vi "saveDataNodeBegin.vi"(8 "error in (no error)":errorcluster, 9 "indent":i32, 10 "XML Refnum in":refnum<file>, 11 "Category in":refnum<class "Category.lvclass">) -> (0 "error out":errorcluster, 2 "XML Refnum out":refnum<file>, 3 "Category out":refnum<class "Category.lvclass">)   [LabVIEW 2013, in "Category.lvclass"]
doc: "Begins the process of saving a xceData Node to an XML formatted file."
uses:
  Category.lvclass
  xCE/xceDataNode/xceDataNode.lvclass
  Category.lvclass/Category.ctl
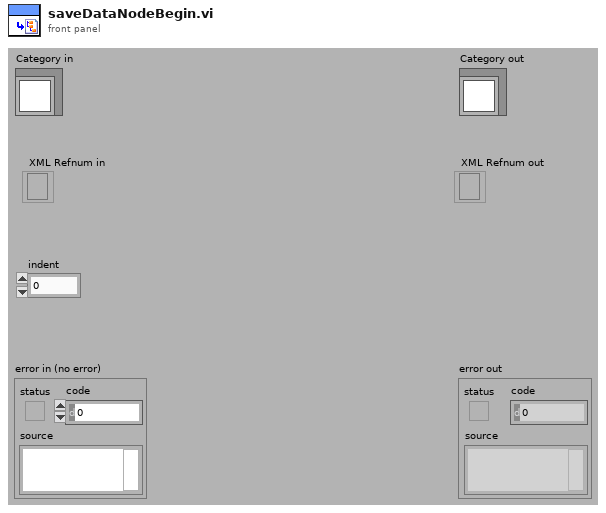
[diagram p1: front panel]
types:
  T1 = typedef "enum_Symbols.ctl" = enum16{"Default", "Analog Input", "Analog Output", "Digital Input", "Digital Output", "PWM Input", "PWM Output"}
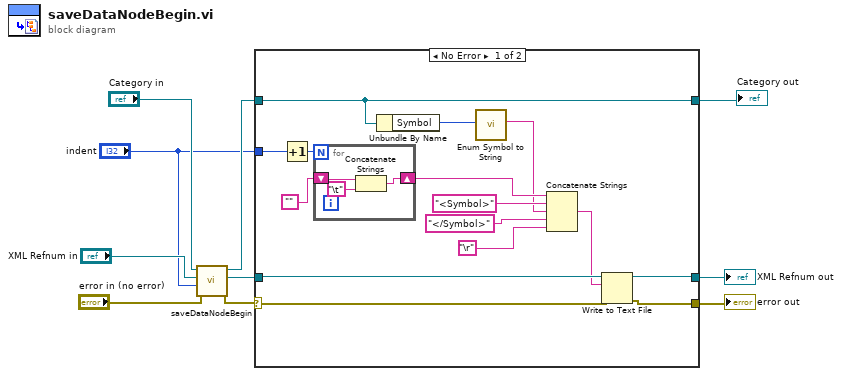
[diagram p0: block diagram]
diagram:
  n1 = call-parent "saveDataNodeBegin.vi"("error in (no error)"="error in (no error)", "indent"="indent", "XML Refnum in"="XML Refnum in", "xceDataNode in"="Category in") -> ("error out"=w7:errorcluster, "XML Refnum out"=w2:refnum<file>, "xceDataNode out"=w6:refnum<class "Category.lvclass">)  [unwired: 5 in]
  n2 = case shown="No Error" w7 {
    selector: w7 -> [w16 w30]
    tunnel: w6 -> [w25 w31]
    tunnel: [w25 w31] -> w5
    tunnel: [w13 w30] -> w4
    tunnel: [w17 w29] -> w3
    tunnel: w2 -> [w15 w29]
    tunnel: "indent" -> [w24 _]
    frame No Error {
      n3 = Increment(x=w24) -> (x+1=w22:i32)
      n4 = for {
        N: w22 -> [_]
        shift-right: [w26] -> w21
        shift-left: "" -> [w28]
        n5 = Concatenate Strings(w28, "\t") -> (w26:string)
      }
      n6 = Unbundle By Name(w25) -> ("Symbol"=w12:T1)
      n7 = call "Enum Symbol to String.vi"("Symbol Enum In"=w12) -> ("Symbol String Out"=w11:string)  [unwired: 10 in]
      n8 = Concatenate Strings(w21, "<Symbol>" ("string"), w11, "</Symbol>" ("string"), "\r") -> (w14:string)
      n9 = Write to Text File(file (use dialog)=w15, text=w14, error in=w16) -> (refnum out=w17:refnum<file>, error out=w13:errorcluster)  [unwired: 1 in, 1 out]
    }
    frame Error {
    }
  }
  "error out" <- w4
  "Category out" <- w5
  "XML Refnum out" <- w3
